vi "Error.Check_Clear Error.vi"(8 "error in (no error)":errorcluster, 10 "Desc":string[](array[string]), 11 "Contains(F)/Match(T)":bool) -> (0 "error out":errorcluster)   [LabVIEW 2024, in "EQMF.lvlib" / "Errors.lvlib"]
uses:
  Errors.lvlib
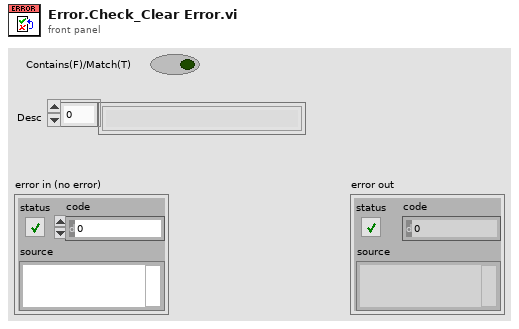
[diagram p1: front panel]
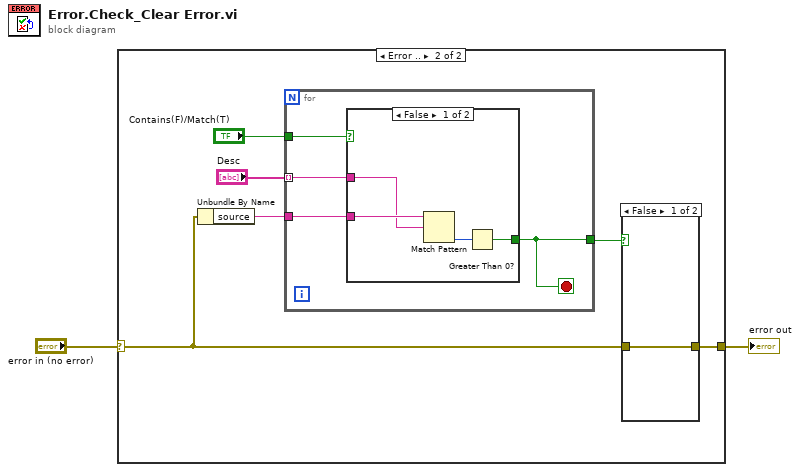
[diagram p0: block diagram]
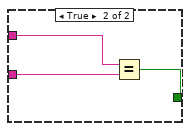
[diagram p4: hidden frame]
diagram:
  n1 = case shown="Error .." "error in (no error)" {
    selector: "error in (no error)" -> [_ w4]
    tunnel: [_ w3] -> w1
    frame No Error {
    }
    frame Error {
      n2 = Unbundle By Name(w4) -> ("source"=w8:string)
      n3 = for {
        tunnel: w8 -> [w13]
        tunnel: "Desc" -> [w11] mode=indexing
        tunnel: "Contains(F)/Match(T)" -> [w12]
        tunnel: [w10] -> w5
        stop <- w10 stop-if-true
        n4 = case shown="False" w12 {
          tunnel: w11 -> [w16 w20]
          tunnel: w13 -> [w17 w19]
          tunnel: [w14 w18] -> w10
          frame False {
            n5 = Match Pattern(string=w17, regular expression=w16) -> (offset past match=w15:i32)  [unwired: 1 in, 3 out]
            n6 = Greater Than 0?(x=w15) -> (x > 0?=w14:bool)
          }
          frame True {
            n7 = Equal?(x=w20, y=w19) -> (x = y?=w18:bool)
          }
        }
      }
      n8 = case shown="False" w5 {
        tunnel: w4 -> [w9 _]
        tunnel: [w9 _] -> w3
        frame False {
        }
        frame True {
        }
      }
    }
  }
  "error out" <- w1
